vi "File IO operation status.vi"(0 "check if valid path (Specify File Path)":bool, 1 "Cancelled by User? (status from a previous dialog)":bool, 5 "File Path":path, 7 "check if valid extension (Specify Extension Type)":bool, 9 "expected extension type":string, 11 "error in (no error)":errorcluster) -> (4 "File Operation Status":T1, 15 "error out":errorcluster)   [LabVIEW 2017]
doc: "SciScan 1.2 160622"
uses:
  File Operation Status.ctl
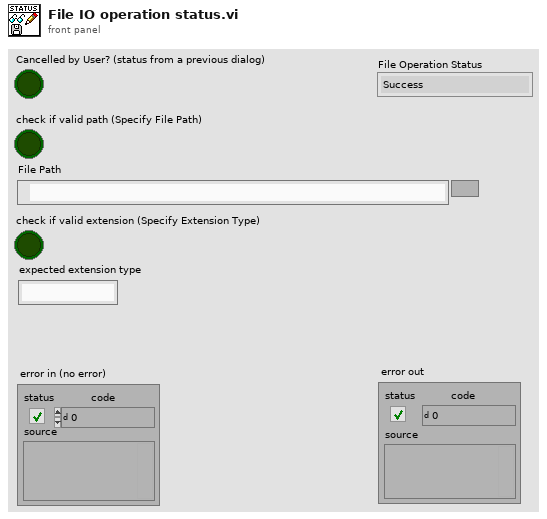
[diagram p1: front panel]
types:
  T1 = typedef "File Operation Status.ctl" = enum16{"Success", "File does not exist", "Cancelled by User", "Incorrect extension type"}
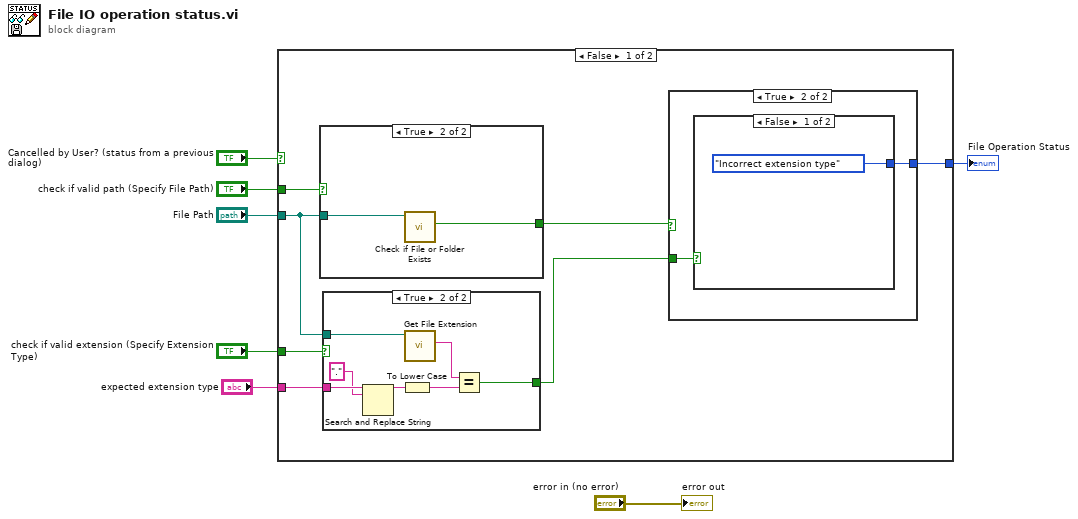
[diagram p0: block diagram]
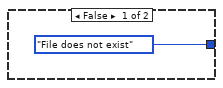
[diagram p2: hidden frame]
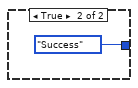
[diagram p3: hidden frame]
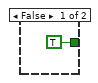
[diagram p4: hidden frame]
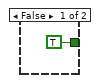
[diagram p5: hidden frame]
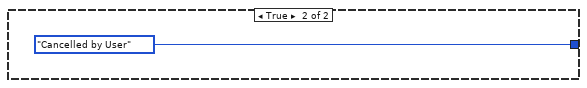
[diagram p6: hidden frame]
diagram:
  n1 = case shown="False" "Cancelled by User? (status from a previous dialog)" {
    tunnel: [w8 File_Operation_Status."Cancelled by User" ("File Operation Status")] -> w6
    tunnel: "check if valid path (Specify File Path)" -> [w14 _]
    tunnel: "File Path" -> [w12 _]
    tunnel: "check if valid extension (Specify Extension Type)" -> [w13 _]
    tunnel: "expected extension type" -> [w11 _]
    frame False {
      n2 = case shown="True" w14 {
        tunnel: w12 -> [_ w30]
        tunnel: [TRUE ("file or folder exists?") w29] -> w10
        frame False {
        }
        frame True {
          n3 = call <vilib>:"Check if File or Folder Exists.vi"("path"=w30) -> ("file or folder exists?"=w29:bool)  [unwired: 8 in, 2 out]
        }
      }
      n4 = case shown="True" w13 {
        tunnel: w12 -> [_ w26]
        tunnel: w11 -> [_ w23]
        tunnel: [TRUE w21] -> w9
        frame False {
        }
        frame True {
          n5 = Search and Replace String(input string=w23, search string=".") -> (result string=w24:string)  [unwired: 6 in, 3 out]
          n6 = To Lower Case(string=w24) -> (all lower case string=w25:string)
          n7 = call <vilib>:"Get File Extension.vi"("file"=w26) -> ("lowercase file extension"=w27:string)  [unwired: 6 in, 4 out]
          n8 = Equal?(x=w27, y=w25) -> (x = y?=w21:bool)
        }
      }
      n9 = case shown="True" w10 {
        tunnel: w9 -> [_ w17]
        tunnel: [File_Operation_Status."File does not exist" ("File Operation Status") w16] -> w8
        frame False {
        }
        frame True {
          n10 = case shown="False" w17 {
            tunnel: [File_Operation_Status."Incorrect extension type" ("File Operation Status") File_Operation_Status."Success" ("File Operation Status")] -> w16
            frame False {
            }
            frame True {
            }
          }
        }
      }
    }
    frame True {
    }
  }
  "File Operation Status" <- w6
  "error out" <- "error in (no error)"
